vi "Init Obj From Cnfg File.vi"(8 "error in (no error)":errorcluster, 10 "Card Config":T1={"Logical Name"="", "Base Settings"={"Clock Source"=1, " clock modulo"=1000000, "TriggerEnabled?"=TRUE, "trigger modulo "=0, "InputTerminated?"=FALSE, "Inhibit(µs)"=1.0, "TriggerLevel"=1.0, "PresetValue"=0, "InternalTrigger?"=FALSE, "InternalArm?"=FALSE, "SWTrigger?"=FALSE, "RisingEdge?"=FALSE, "StopOnPreset?"=FALSE, "ResetWhenDone?"=TRUE, "Gate Divider"=1, "PositiveGate?"=TRUE}, "SG08_Settings"={"Gate Terminate"=TRUE, "Gate Level"=1.0, "Gate Delay (µs)"=0.0, "StepBackTime (µs)"=0.0, "Burst Counter"=0, "Trigger Divider"=1, "Trigger Multiplier"=4}, "Channel Names"=[], "Advanced Settings"={"Trigger on MS Bus"=24, "Force Trigger (µs)"=0.0, "Gate Type"=TRUE, "Synchronize Gate"=FALSE}} {"Advanced Settings"."Trigger on MS Bus" format="%04x" items=["Local Primary0x1"=1, "Local Secondary0x2"=2, "Local Force 0x4"=4, "Resynchronize 0x8"=8, "Master Prim. 0x10"=16, "Master Sec. 0x20"=32, "Master Force  0x40"=64, "System Clock 0x80"=128, "Delay Clock 0x100"=256, "Inhibit Local 0x200"=512, "Start Local 0x400"=1024, "Start Bus 0x800"=2048, "Step Back Local 0x1000"=4096, "Step Back Bus 0x2000"=8192, "RunCircle 0x4000"=16384, "SyncReload 0x8000"=32768, "From E 0x10000"=65536, "From F 0x20000"=131072, "From Bus 0x40000"=262144]; "Advanced Settings"."Force Trigger (µs)" min=0.0 format="%.6f"; "SG08_Settings"."StepBackTime (µs)" min=0.0 format="%.6f"; "SG08_Settings"."Gate Delay (µs)" format="%.3f"; "SG08_Settings"."Gate Level" min=-2.5 max=2.5 format="%.3g"; "Base Settings"."Gate Divider" min=1 max=1000000; "Base Settings"."Clock Source" items=["Internal Oscillator"=1, "External Trigger"=2, "Trigger-> Oscillator"=3, "MasterSlave Bus"=4]; "Base Settings"."Inhibit(µs)" format="%#_11g"}, 11 "BME_DG_Base in":refnum<class "BME_DG_Base.lvclass">) -> (0 "error out":errorcluster, 3 "BME_DG_Base out":refnum<class "BME_DG_Base.lvclass">)   [LabVIEW 2009, in "POLARIS BME DG.lvlib" / "BME_DG_Base.lvclass"]
uses:
  BME_DG_Base.lvclass
  Card Config.ctl
  LV-BME Interface/BME_DG_TriggerSettings.ctl
  LV-BME Interface/ClockSource.ctl
  SG08_Settings.ctl
  LV-BME Interface/BME_DG_V2TriggerSettings.ctl
  MSBus.ctl
  BME_DG_Chnl/BME_DG_Chnl.lvclass
  POLARIS BME DG.lvlib
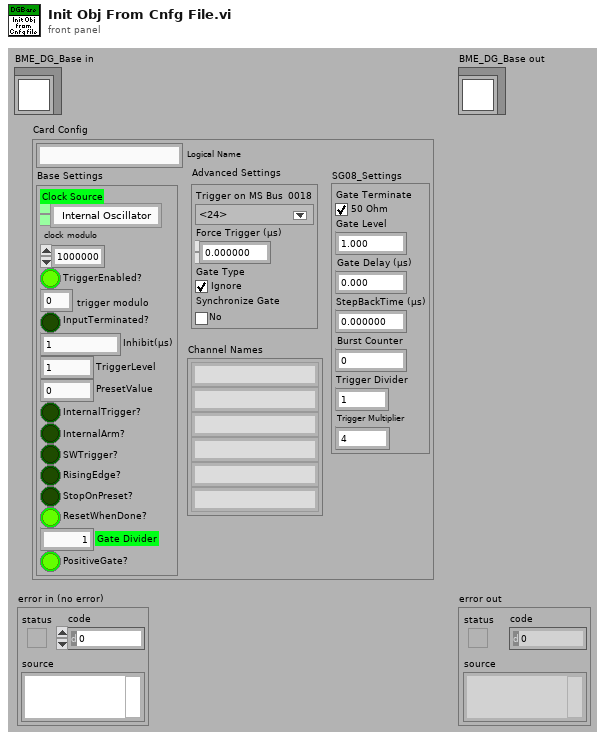
[diagram p1: front panel]
types:
  T1 = typedef "POLARIS BME DG.lvlib/Card Config.ctl" = cluster{"Logical Name":string, "Base Settings":T2, "SG08_Settings":T4, "Channel Names":string[], "Advanced Settings":T5}
  T2 = typedef "POLARIS BME DG.lvlib/BME_DG_TriggerSettings.ctl" = cluster{"Clock Source":T3, " clock modulo":u32, "TriggerEnabled?":bool, "trigger modulo ":i32, "InputTerminated?":bool, "Inhibit(µs)":dbl, "TriggerLevel":dbl, "PresetValue":i32, "InternalTrigger?":bool, "InternalArm?":bool, "SWTrigger?":bool, "RisingEdge?":bool, "StopOnPreset?":bool, "ResetWhenDone?":bool, "Gate Divider":i32, "PositiveGate?":bool}
  T3 = typedef "POLARIS BME DG.lvlib/ClockSource.ctl" = i32
  T4 = typedef "POLARIS BME DG.lvlib/SG08_Settings.ctl" = cluster{"Gate Terminate":bool, "Gate Level":dbl, "Gate Delay (µs)":dbl, "StepBackTime (µs)":dbl, "Burst Counter":u32, "Trigger Divider":u32, "Trigger Multiplier":u32}
  T5 = typedef "POLARIS BME DG.lvlib/BME_DG_V2TriggerSettings.ctl" = cluster{"Trigger on MS Bus":T6, "Force Trigger (µs)":dbl, "Gate Type":bool, "Synchronize Gate":bool}
  T6 = typedef "POLARIS BME DG.lvlib/MSBus.ctl" = u32
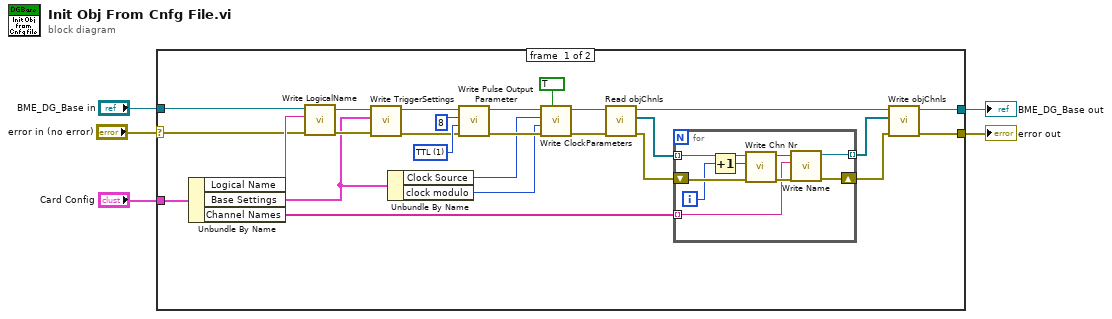
[diagram p0: block diagram]
diagram:
  n1 = case shown="No Error" "error in (no error)" {
    selector: "error in (no error)" -> [w15 w42]
    tunnel: [w14 w42] -> w4
    tunnel: [w21 w41] -> w2
    tunnel: "BME_DG_Base in" -> [w30 w41]
    tunnel: "Card Config" -> [w31 _]
    frame #0 {
      w25 = u32 1 items=["TTL"=1, "NIM"=2, "ECL"=3] ("Pulse Output Level")
      n2 = Unbundle By Name(w31) -> ("Logical Name"=w29:string, "Base Settings"=w8:T2, "Channel Names"=w18:string[])
      n3 = call "Write LogicalName.vi"("error in (no error)"=w15, "LogicalName"=w29, "BME_DG_Base in"=w30) -> ("error out"=w27:errorcluster, "BME_DG_Base out"=w28:refnum<class "BME_DG_Base.lvclass">)  [unwired: 7 in]
      n4 = call-dynamic "Write TriggerSettings.vi"("error in (no error)"=w27, "Trigger Settings"=w8, "BME_DG_Base in"=w28) -> ("error out"=w24:errorcluster, "BME_DG_Base out"=w23:refnum<class "BME_DG_Base.lvclass">)  [unwired: 7 in]
      n5 = Unbundle By Name(w8) -> ("Clock Source"=w7:T3, "clock modulo"=w6:u32)
      n6 = call-dynamic "Write Pulse Output Parameter.vi"("error in (no error)"=w24, "Pulse Output Level"=w25, "Pulse Width"=u32 8, "BME_DG_Base in"=w23) -> ("error out"=w10:errorcluster, "BME_DG_Base out"=w12:refnum<class "BME_DG_Base.lvclass">)  [unwired: 6 in]
      n7 = call-dynamic "Write ClockParameters.vi"("ClockEnable"=TRUE, "error in (no error)"=w10, "PrescalerCrystalOscilator"=w6, "ClockSource"=w7, "BME_DG_Base in"=w12) -> ("error out"=w9:errorcluster, "BME_DG_Base out"=w11:refnum<class "BME_DG_Base.lvclass">)  [unwired: 5 in]
      n8 = call-dynamic "Read objChnls.vi"("error in (no error)"=w9, "BME_DG_Base in"=w11) -> ("error out"=w17:errorcluster, "objChnls"=w20:refnum<class "BME_DG_Chnl.lvclass">[], "BME_DG_Base out"=w22:refnum<class "BME_DG_Base.lvclass">)  [unwired: 6 in, 1 out]
      n9 = for {
        tunnel: w20 -> [w40] mode=indexing
        shift-right: [w34] -> w16
        shift-left: w17 -> [w38]
        tunnel: [w33] -> w19 mode=indexing
        tunnel: w18 -> [w32] mode=indexing
        i -> [w35]
        n10 = Increment(x=w35) -> (x+1=w36:i32)
        n11 = call-dynamic "Write Chn Nr.vi"("error in (no error)"=w38, "Chn Nr"=w36, "BME_DG_Chnl in"=w40) -> ("error out"=w37:errorcluster, "BME_DG_Chnl out"=w39:refnum<class "BME_DG_Chnl.lvclass">)  [unwired: 7 in]
        n12 = call-dynamic "Write Name.vi"("error in (no error)"=w37, "Name"=w32, "BME_DG_Chnl in"=w39) -> ("error out"=w34:errorcluster, "BME_DG_Chnl out"=w33:refnum<class "BME_DG_Chnl.lvclass">)  [unwired: 7 in]
      }
      n13 = call-dynamic "Write objChnls.vi"("error in (no error)"=w16, "objChnls"=w19, "BME_DG_Base in"=w22) -> ("error out"=w14:errorcluster, "BME_DG_Base out"=w21:refnum<class "BME_DG_Base.lvclass">)  [unwired: 7 in]
    }
    frame #1 {
    }
  }
  "error out" <- w4
  "BME_DG_Base out" <- w2
